vi "Close Logger.vi"(8 "error in (no error)":errorcluster, 11 "Logger in.lvclass":refnum<class "Logger.lvclass">) -> (0 "error out":errorcluster)   [LabVIEW 2017, in "Logger.lvclass"]
uses:
  Logger.lvclass
  Logger.lvclass/Logger.ctl
  <vilib>/TagLibrary/Close Tag (Single).vi
  <vilib>/Message/Close (Sync).vi
  <vilib>/TagLibrary/TagLibrary.lvlib
  <vilib>/Message/Message.lvlib
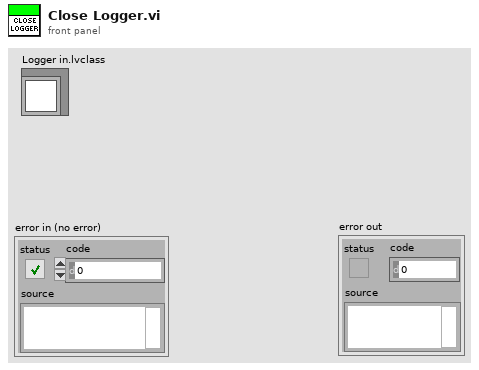
[diagram p1: front panel]
types:
  T1 = cluster{"Tag Reference":refnum<k21>, "Tag Units":string, "Tag Path":string, "Waveform":waveform(dbl), "Log":bool}[]
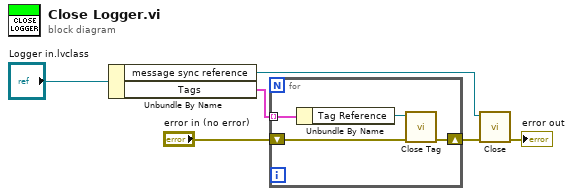
[diagram p0: block diagram]
diagram:
  n1 = Unbundle By Name("Logger in.lvclass") -> ("message sync reference"=w2:refnum<k21>, "Tags"=w1:T1)
  n2 = for {
    tunnel: w1 -> [w10] mode=indexing
    shift-right: [w7] -> w3
    shift-left: "error in (no error)" -> [w8]
    n3 = Unbundle By Name(w10) -> ("Tag Reference"=w9:refnum<k21>)
    n4 = call-poly <vilib>:"Close Tag.vi"("error in (no error)"=w8, "tag reference"=w9) -> ("error out"=w7:errorcluster)  [unwired: 9 in]
  }
  n5 = call-poly <vilib>:"Close.vi"("error in"=w3, "message sync reference"=w2) -> ("error out"=→"error out":errorcluster)  [unwired: 9 in]
